vi "Build folder file path.vi"(8 "error in (no error)":errorcluster, 9 "File name":string="HPLC data", 10 "Folder name":string="HPLC data", 11 "Experiment file path":path) -> (0 "error out":errorcluster, 3 "Path":path)   [LabVIEW 2017]
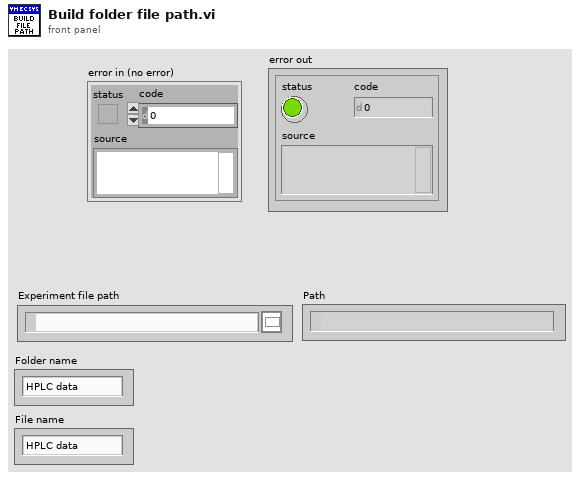
[diagram p1: front panel]
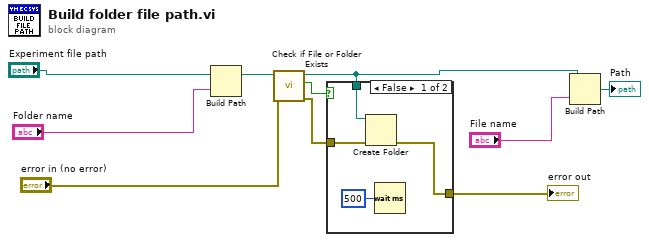
[diagram p0: block diagram]
diagram:
  n1 = Build Path(base path="Experiment file path", name or relative path="Folder name") -> (appended path=w4:path)
  n2 = call <vilib>:"Check if File or Folder Exists.vi"("error in (no error)"="error in (no error)", "path"=w4) -> ("error out"=w7:errorcluster, "file or folder exists?"=w8:bool)  [unwired: 7 in, 1 out]
  n3 = case shown="False" w8 {
    tunnel: w4 -> [w13 _]
    tunnel: w7 -> [w11 w14]
    tunnel: [w10 w14] -> w1
    frame False {
      n4 = Create Folder(path (use dialog)=w13, error in=w11) -> (error out=w10:errorcluster)  [unwired: 1 in, 2 out]
      n5 = Wait (ms)(milliseconds to wait=u32 500) -> ()  [unwired: 1 out]
    }
    frame True {
    }
  }
  "error out" <- w1
  n6 = Build Path(base path=w4, name or relative path="File name") -> (appended path=→"Path":path)
